vi "Configure Measurements (Normal).vi"(8 "error in (no error)":errorcluster, 10 "Normal Measurements":i32[](listbox)=[0, 1, 2, 3, 4, 5, 6], 11 "VISA resource name":refnum<visa-resource-name>) -> (0 "error out":errorcluster, 3 "VISA resource name out":refnum<visa-resource-name>)   [LabVIEW 2015, in "Voltech PM1000+.lvlib"]
doc: "Configures the operating mode, measurement itmes. This vi can only be used when PM1000+ is set to Normal mode by using \"Configure Mode\" vi."
uses:
  <instrlib>/Voltech PM1000+/Voltech PM1000+.lvlib
panel:
  # "Notice:  \nHold \"Ctrl\" key and click the \nmeasurements to select \nmultiple items."
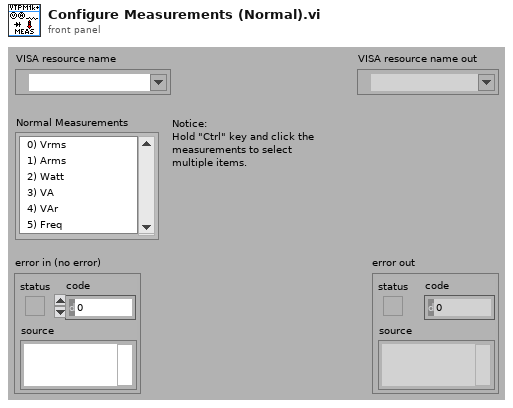
[diagram p1: front panel]
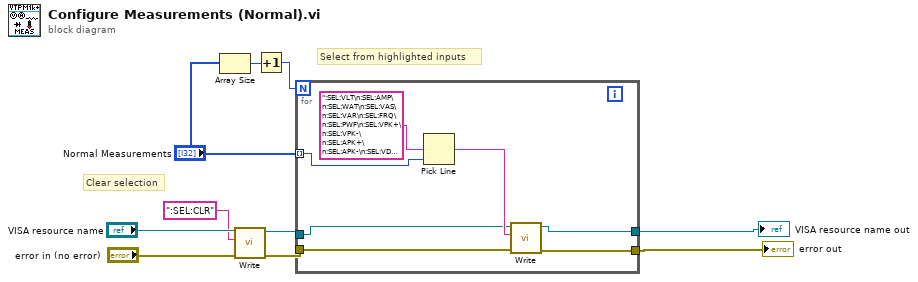
[diagram p0: block diagram]
diagram:
  # "Select from highlighted inputs"
  # "Clear selection"
  n1 = Array Size(array="Normal Measurements") -> (size(s)=w9:i32)
  n2 = call <instrlib>:"Write.vi"("error in (no error)"="error in (no error)", "Write Buffer"=":SEL:CLR" ("multi-line string"), "VISA resource name"="VISA resource name") -> ("error out"=w3:errorcluster, "VISA resource name out"=w4:refnum<visa-resource-name>)  [unwired: 7 in]
  n3 = Increment(x=w9) -> (x+1=w8:i32)
  n4 = for {
    N: w8 -> [_]
    tunnel: "Normal Measurements" -> [w16] mode=indexing
    tunnel: [w15] -> w2
    tunnel: [w14] -> w1
    tunnel: w4 -> [w12]
    tunnel: w3 -> [w11]
    n5 = Pick Line(multi-line string=":SEL:VLT\n:SEL:AMP\n:SEL:WAT\n:SEL:VAS\n:SEL:VAR\n:SEL:FRQ\n:SEL:PWF\n:SEL:VPK+\n:SEL:VPK-\n:SEL:APK+\n:SEL:APK-\n:SEL:VDC\n:SEL:ADC\n:SEL:VCF\n:SEL:ACF\n:SEL:VDF\n:SEL:ADF\n:SEL:IMP\n:SEL:RES\n:SEL:REA\n:SEL:VHM\n:SEL:AHM\n:SEL:VRNG\n:SEL:ARNG", line index=w16) -> (output string=w13:string)  [unwired: 1 in]
    n6 = call <instrlib>:"Write.vi"("error in (no error)"=w11, "Write Buffer"=w13, "VISA resource name"=w12) -> ("error out"=w14:errorcluster, "VISA resource name out"=w15:refnum<visa-resource-name>)  [unwired: 7 in]
  }
  "error out" <- w1
  "VISA resource name out" <- w2
